vi "Test Broadcast Init.vi"(8 "error in (no error)":errorcluster, 11 "TestCase in":refnum<class "Test Module Init.lvclass">) -> (0 "error out":errorcluster, 3 "TestCase out":refnum<class "Test Module Init.lvclass">)   [LabVIEW 2020, in "Test Module Init.lvclass"]
uses:
  Test Module Init.lvclass
  <vilib>/addons/_JKI Toolkits/VI Tester/TestCase.llb/TestCase.lvclass
  Libraries/Osciloscope/Osciloscope.lvlib
  C:/Program Files (x86)/National Instruments/LabVIEW 2020/vi.lib/addons/_JKI Toolkits/VI Tester/TestCase.llb/TestCase.lvclass
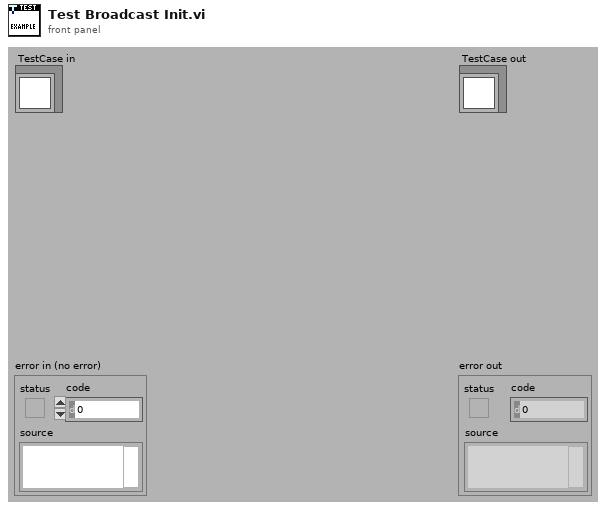
[diagram p1: front panel]
types:
  T1 = typedef "Osciloscope.lvlib/Broadcast Events--cluster.ctl" = cluster{"Module Did Init":refnum<user-event>, "Status Updated":refnum<user-event>, "Error Reported":refnum<user-event>, "Module Did Stop":refnum<user-event>, "Update Module Execution Status":refnum<user-event>, "Obtain Osciloscope Name":refnum<user-event>}
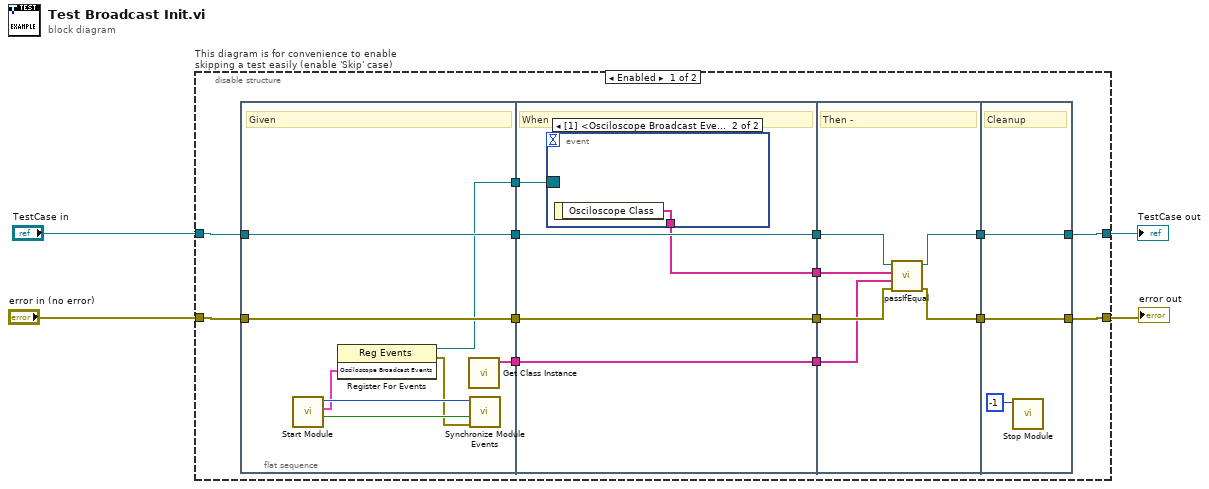
[diagram p0: block diagram]
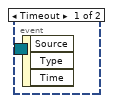
[diagram p2: hidden frame]
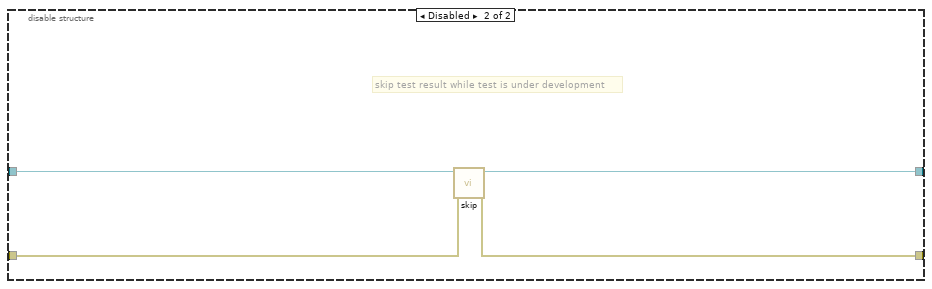
[diagram p3: hidden frame]
diagram:
  n1 = disable-structure "This diagram is for convenience to enable skipping a test easily (enable 'Skip' case)" shown="Enabled" {
    disable-tunnel: "TestCase in" -> [w12 w45]
    disable-tunnel: [w10 w43] -> w1
    disable-tunnel: [w9 w44] -> w3
    disable-tunnel: "error in (no error)" -> [w11 w42]
    frame Enabled {
      n2 = flat-sequence {
        tunnel: w11 -> [w25]
        tunnel: w12 -> [w26]
        tunnel: [w26] -> w18
        tunnel: [w25] -> w17
        tunnel: [w20] -> w8
        tunnel: [w19] -> w5
        tunnel: [w31] -> w16
        tunnel: [w30] -> w15
        tunnel: w18 -> [w31]
        tunnel: w17 -> [w30]
        tunnel: w8 -> [w29]
        tunnel: [w28] -> w7
        tunnel: [w27] -> w6
        tunnel: w5 -> [w27]
        tunnel: [w37] -> w14
        tunnel: [w35] -> w13
        tunnel: w16 -> [w38]
        tunnel: w15 -> [w36]
        tunnel: w7 -> [w34]
        tunnel: w6 -> [w33]
        tunnel: [w40] -> w9
        tunnel: [w41] -> w10
        tunnel: w14 -> [w41]
        tunnel: w13 -> [w40]
        frame #0 {
          # "Given"
          n3 = call "Start Module.vi"() -> ("Wait for Event Sync?"=w24:bool, "Osciloscope Broadcast Events"=w22:T1, "Module ID"=w23:i32)  [unwired: 8 in, 1 out]
          n4 = register-events(w22) -> (reference out=w20:refnum<event-registration>, error out=w21:errorcluster)  [unwired: 2 in]
          n5 = call "Get Class Instance.vi"() -> ("Classes"=w19:string[])  [unwired: 11 in]
          n6 = call "Synchronize Module Events.vi"("error in"=w21, "Wait for Event Sync?"=w24, "Module ID in"=w23) -> ()  [unwired: 7 in, 2 out]
        }
        frame #1 {
          # "When -"
          n7 = event shown="[1] <Osciloscope Broadcast Events.Obtain Osciloscope Name>: User Event" {
            selector: w29 -> [_ _]
            dyn-events: _ -> [_ _]
            timeout: _ -> [_ _]
            tunnel: [_ w32] -> w28
            event Timeout {
              n8 = event-data() -> ()  [unwired: 1 in, 3 out]
            }
            event User Event {
              n9 = event-data() -> ("Osciloscope Class"=w32:string[])  [unwired: 1 in]
            }
          }
        }
        frame #2 {
          # "Then -"
          n10 = call-dynamic "passIfEqual.vi"("error in (no error)"=w36, "y"=w33, "x"=w34, "TestCase in"=w38) -> ("error out"=w35:errorcluster, "TestCase out"=w37:refnum<class "Test Module Init.lvclass">)  [unwired: 6 in]
        }
        frame #3 {
          # "Cleanup"
          n11 = call "Stop Module.vi"("Module ID"=-1) -> ()  [unwired: 10 in, 1 out]
        }
      }
    }
    frame Disabled {
      # "skip test result while test is under development"
      n12 = call <vilib>:"skip.vi"("error in (no error)"=w42, "TestCase in"=w45) -> ("error out"=w44:errorcluster, "TestCase out"=w43:refnum<class "Test Module Init.lvclass">)  [unwired: 8 in]
    }
  }
  "error out" <- w3
  "TestCase out" <- w1
